vi "Defer Updates.vi"(8 "Error In":errorcluster, 11 "Panel Actor in":refnum<class "Panel Actor.lvclass">) -> (0 "Error Out":errorcluster, 2 "Deferer":refnum<class "Deferer.lvclass">)   [LabVIEW 2019, in "Panel Actor.lvlib" / "Panel Actor.lvclass"]
doc: "Defers updates for the panel.\n\n<B>Controller In:</B> Panel Helper object to handle Defer\n<B>Error In:</B> Describes error conditions that occur before this node runs.\n\n<B>Deferer:</B> Deferer object.\n<B>Error Out:</B> Contains error information.\n----\nPlease see the following web address for additional documentation and tutorial information:\nhttp://www.mooregoodideas.com/mgi-panel-manager/\n\nAuthor: Derek Trepanier\n\nCopyright (c) 2018, Moore Good Ideas, Inc.\n\nAll rights reserved.\n\nRedistribution and use in source and binary forms, with or without modification, are permitted provided that the following conditions are met:\n\n * Redistributions of source code must retain the above copyright notice, this list of conditions and the following disclaimer.\n * Redistributions in binary form must reproduce the above copyright notice, this list of conditions and the following disclaimer in the documentation and/or other materials provided with the distribution.\n * Neither the name of Moore Good Ideas, Inc. nor the names of its contributors may be used to endorse or promote products derived from this software without specific prior written permission.\n\nTHIS SOFTWARE IS PROVIDED BY THE COPYRIGHT HOLDERS AND CONTRIBUTORS \"AS IS\" AND ANY EXPRESS OR IMPLIED WARRANTIES, INCLUDING, BUT NOT LIMITED TO, THE IMPLIED WARRANTIES OF MERCHANTABILITY AND FITNESS FOR A PARTICULAR PURPOSE ARE DISCLAIMED. IN NO EVENT SHALL THE COPYRIGHT OWNER OR CONTRIBUTORS BE LIABLE FOR ANY DIRECT, INDIRECT, INCIDENTAL, SPECIAL, EXEMPLARY, OR CONSEQUENTIAL DAMAGES (INCLUDING, BUT NOT LIMITED TO, PROCUREMENT OF SUBSTITUTE GOODS OR SERVICES; LOSS OF USE, DATA, OR PROFITS; OR BUSINESS INTERRUPTION) HOWEVER CAUSED AND ON ANY THEORY OF LIABILITY, WHETHER IN CONTRACT, STRICT LIABILITY, OR TORT (INCLUDING NEGLIGENCE OR OTHERWISE) ARISING IN ANY WAY OUT OF THE USE OF THIS SOFTWARE, EVEN IF ADVISED OF THE POSSIBILITY OF SUCH DAMAGE."
uses:
  Panel Actor.lvclass
  builds/Engine/Panel.lvlibp/Panel Helper/Panel Helper.lvclass
  builds/Engine/Panel.lvlibp/Deferer/Deferer.lvclass
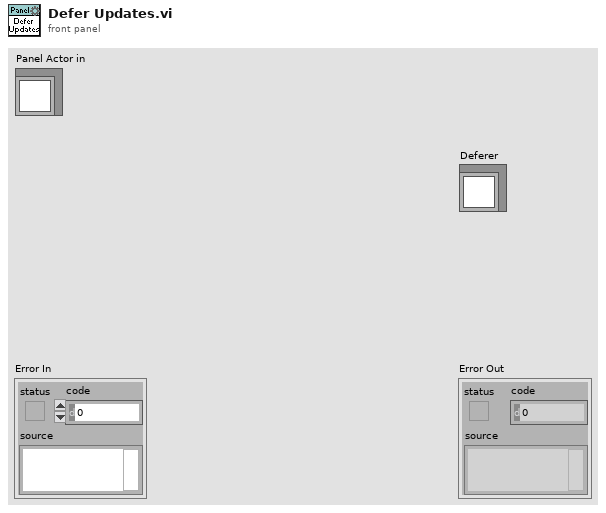
[diagram p1: front panel]
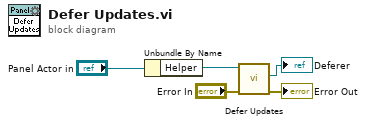
[diagram p0: block diagram]
diagram:
  n1 = Unbundle By Name("Panel Actor in") -> ("Helper"=w4:refnum<class "Panel Helper.lvclass">)
  n2 = call "Defer Updates.vi"("Error In"="Error In", "Controller in"=w4) -> ("Error Out"=→"Error Out":errorcluster, "Deferer"=→"Deferer":refnum<class "Deferer.lvclass">)  [unwired: 8 in]
